vi "PS (single).vi"(8 "error in (no error)":errorcluster, 11 "XY-data":cluster{"X-array":dbl[], "Y-array":dbl[]} {"Y-array" format="%.2p"; "X-array" format="%.2p"}) -> (0 "error out":errorcluster, 2 "Power Spectrum":cluster{"f0":dbl, "df":dbl, "magnitude":dbl[]} {"magnitude" format="%.2p"; "f0" format="%0.2p"; "df" format="%0.2p"}, 3 "XY-data out":cluster{"X-array":dbl[], "Y-array":dbl[]} {"Y-array" format="%.2p"; "X-array" format="%.2p"})   [LabVIEW 2016, in "xy_utilities.lvlib"]
doc: "Computes the Power Spectrum of <B>XY-data</B>. This VI is a wrapper for NI_MAPro.lvlib:FFT Power Spectrum and PSD.vi.\n\nWire data to the data input to determine the polymorphic instance to use or manually select the instance."
uses:
  xy_utilities.lvlib
  <vilib>/measure/maspectr.llb/Power Spectrum and PSD Export Mode.ctl
  Sort (single).vi
  <vilib>/measure/maresamp.llb/Resample Pair of Arrays (single shot).vi
  <vilib>/measure/maspectr.llb/FFT Power Spectrum and PSD for 1 Chan.vi
  <vilib>/measure/NI_MAPro.lvlib
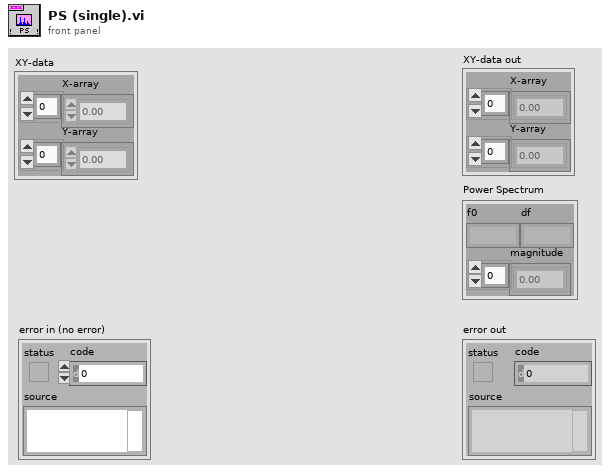
[diagram p1: front panel]
types:
  T1 = typedef "NI_MAPro.lvlib/Power Spectrum and PSD Export Mode.ctl" = u16
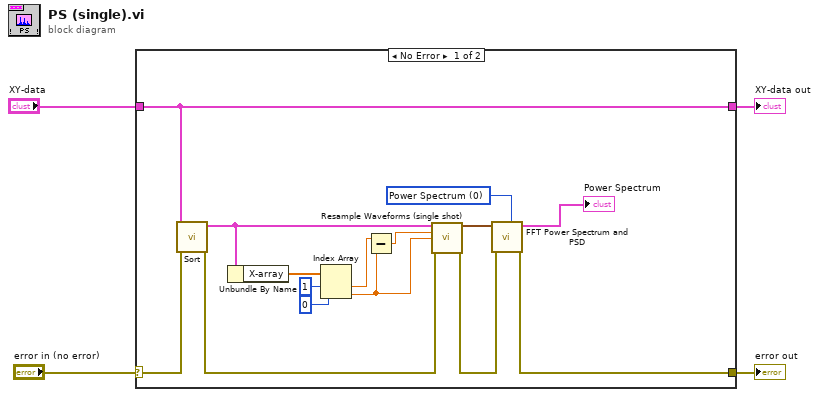
[diagram p0: block diagram]
diagram:
  n1 = case shown="No Error" "error in (no error)" {
    selector: "error in (no error)" -> [w9 w21]
    tunnel: [w6 w21] -> w3
    tunnel: "XY-data" -> [w17 w20]
    tunnel: [w17 w20] -> w1
    frame No Error {
      w5 = T1 0 items=["Power Spectrum", "Power Spectral Density"] ("export mode")
      n2 = call-poly "Sort.vi"("error in (no error)"=w9, "XY-data"=w17) -> ("error out"=w8:errorcluster, "Sorted XY-data out"=w16:cluster{"X-array":dbl[], "Y-array":dbl[]})  [unwired: 8 in]
      n3 = Unbundle By Name(w16) -> ("X-array"=w15:dbl[])
      n4 = Index Array(array=w15, index #1=1 ("index"), index #2=0 ("index")) -> (element #1=w12:dbl, element #2=w11:dbl)
      n5 = Subtract(x=w12, y=w11) -> (x-y=w10:dbl)
      n6 = call-poly <vilib>:"Resample Waveforms (single shot).vi"("XY-data in"=w16, "dt"=w10, "t0"=w11, "error in (no error)"=w8) -> ("resampled waveform out"=w19:waveform(dbl), "error out"=w7:errorcluster)  [unwired: 7 in, 3 out]
      n7 = call-poly <vilib>:"FFT Power Spectrum and PSD.vi"("export mode"=w5, "error in (no error)"=w7, "time signal"=w19) -> ("error out"=w6:errorcluster, "Power Spectrum / PSD"=→"Power Spectrum":cluster{"f0":dbl, "df":dbl, "magnitude":dbl[]})  [unwired: 5 in, 2 out]
    }
    frame Error {
    }
  }
  "error out" <- w3
  "XY-data out" <- w1
